vi "Get Objects greater than.vi"(8 "error in":errorcluster, 10 "Lower Bound":u16 format="%.0x", 11 "Sorted Object Dictionary in":refnum<class "Sorted Object Dictionary.lvclass">) -> (0 "error out":errorcluster, 2 "Entries":refnum<class "OD Entry.lvclass">[](array[class]), 3 "Sorted Object Dictionary out":refnum<class "Sorted Object Dictionary.lvclass">)   [LabVIEW 2020, in "Electronic Datasheet.lvlib" / "Sorted Object Dictionary.lvclass"]
uses:
  Sorted Object Dictionary.lvclass
  Sorted Object Dictionary.lvclass/Sorted Object Dictionary.ctl
  OD Entry/OD Entry.lvclass
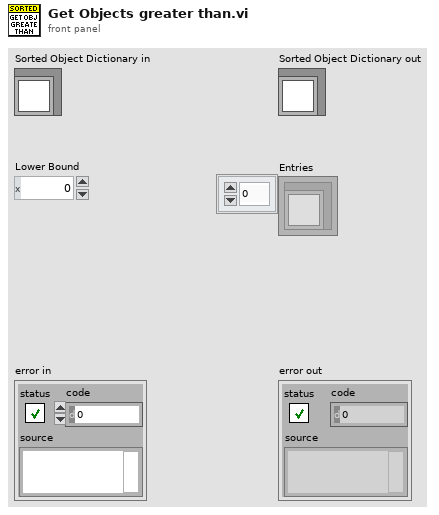
[diagram p1: front panel]
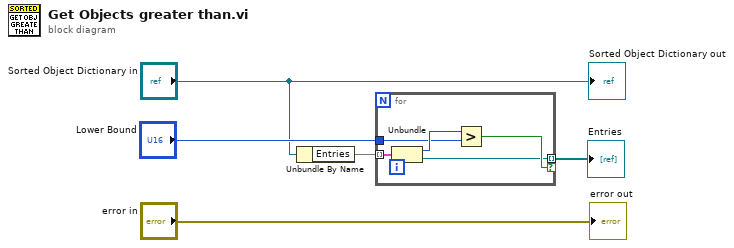
[diagram p0: block diagram]
diagram:
  n1 = Unbundle By Name("Sorted Object Dictionary in") -> ("Entries"=w1:map{u16, refnum<class "OD Entry.lvclass">})
  n2 = for {
    tunnel: w1 -> [w10] mode=indexing
    tunnel: "Lower Bound" -> [w6]
    tunnel: [w8] -> w5 mode=indexing if=w9
    n3 = Unbundle(w10) -> ("Index"=w7:u16, "OD Entry"=w8:refnum<class "OD Entry.lvclass">)
    n4 = Greater?(x=w7, y=w6) -> (0:w9:bool)
  }
  "Entries" <- w5
  "error out" <- "error in"
  "Sorted Object Dictionary out" <- "Sorted Object Dictionary in"
